vi "Read Next Message.vi"(7 "Ignore Error on Termination Message (F)":bool, 8 "error in (no error)":errorcluster, 9 "Termination List ([Exit])":string[](array[string])=["Exit"], 10 "timeout (1ms)":i32=1, 11 "Message Queue in":T3) -> (0 "error out":errorcluster, 1 "Message Value":string, 2 "Message Name":string, 3 "Message Queue out":T3, 4 "Message Attributes":T1, 5 "Exit Process":bool, 6 "Message":T2)   [LabVIEW 2013, in "AMC.lvlib"]
doc: "This VI returns the next message from the message queue passed in. If the returned message matches any of the message names listed in the Termination List the Exit Process indicator will return True. If no message is available on the queue within the Timeout limit, the VI returns with the Timed Out indicator set True."
uses:
  AMC.lvlib
  _SubVIs/TypeDefs/Message Queue.ctl
  _SubVIs/TypeDefs/Message.ctl
  Keyed Array/KeyedArray.ctl
  Keyed Array/Tools_KeyedArray.lvlib
panel:
  out "Timed Out":bool
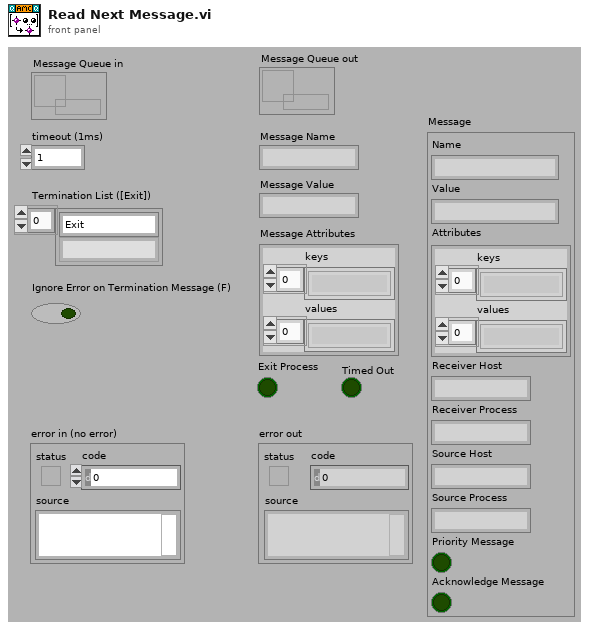
[diagram p1: front panel]
types:
  T1 = typedef "Tools_KeyedArray.lvlib/KeyedArray.ctl" = cluster{"keys":string[], "values":string[]}
  T2 = typedef "AMC.lvlib/Message.ctl" = cluster{"Name":string, "Value":string, "Attributes":T1, "Receiver Host":string, "Receiver Process":string, "Source Host":string, "Source Process":string, "Priority Message":bool, "Acknowledge Message":bool}
  T3 = typedef "AMC.lvlib/Message Queue.ctl" = refnum<queue>
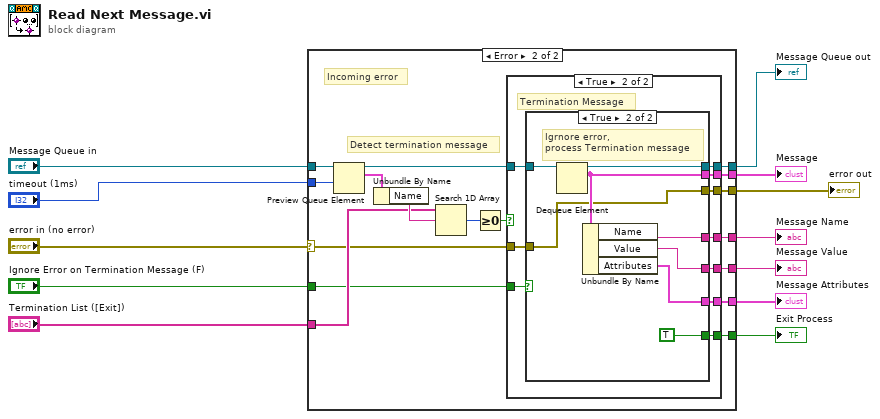
[diagram p0: block diagram]
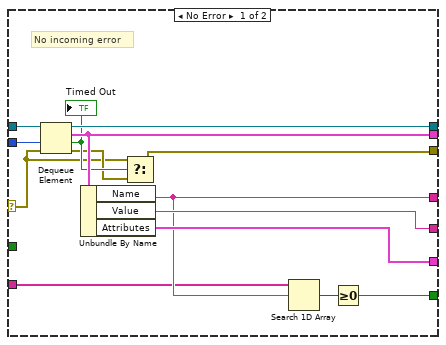
[diagram p2: hidden frame]
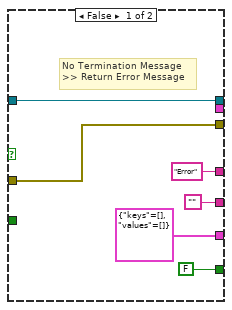
[diagram p3: hidden frame]
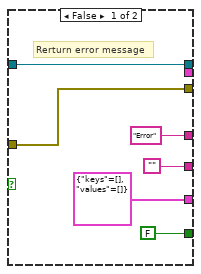
[diagram p4: hidden frame]
diagram:
  n1 = case shown="Error" "error in (no error)" {
    selector: "error in (no error)" -> [w13 w29]
    tunnel: "Message Queue in" -> [w26 w39]
    tunnel: [w25 w31] -> w10
    tunnel: [w20 w43] -> w12
    tunnel: "timeout (1ms)" -> [w24 w38]
    tunnel: [w14 w27] -> w11
    tunnel: [w22 w42] -> w9
    tunnel: [w23 w28] -> w8
    tunnel: [w21 w41] -> w7
    tunnel: "Termination List ([Exit])" -> [w19 w34]
    tunnel: [w17 w40] -> w6
    tunnel: "Ignore Error on Termination Message (F)" -> [_ w30]
    frame No Error {
      # "No incoming error"
      n2 = Dequeue Element(queue=w26, timeout in ms (-1)=w24, error in (no error)=w13) -> (queue out=w25:T3, element=w23:T2, timed out?=w16:bool, error out=w15:errorcluster)
      "Timed Out" <- w16
      n3 = Unbundle By Name(w23) -> ("Name"=w20:string, "Value"=w22:string, "Attributes"=w21:T1)
      n4 = Select(t=w13, s=w16, f=w15) -> (s? t:f=w14:errorcluster)
      n5 = Search 1D Array(1D array=w19, element=w20) -> (index of element=w18:i32)  [unwired: 1 out]
      n6 = Greater Or Equal To 0?(x=w18) -> (x >= 0?=w17:bool)
    }
    frame Error {
      # "Detect termination message"
      # "Incoming error"
      n7 = Preview Queue Element(queue=w39, timeout in ms (-1)=w38) -> (queue out=w32:T3, element=w37:T2)  [unwired: 1 in, 2 out]
      n8 = Unbundle By Name(w37) -> ("Name"=w35:string)
      n9 = Search 1D Array(1D array=w34, element=w35) -> (index of element=w36:i32)  [unwired: 1 out]
      n10 = Greater Or Equal To 0?(x=w36) -> (x >= 0?=w33:bool)
      n11 = case shown="True" w33 {
        tunnel: ["Error" w57] -> w43
        tunnel: ["" w56] -> w42
        tunnel: [T1 {"keys"=[], "values"=[]} ("Attributes") w55] -> w41
        tunnel: [FALSE w54] -> w40
        tunnel: [w45 w53] -> w31
        tunnel: w32 -> [w45 w59]
        tunnel: w30 -> [_ w58]
        tunnel: w29 -> [w44 w50]
        tunnel: [_ w52] -> w28
        tunnel: [w44 w51] -> w27
        frame False {
          # "No Termination Message\n>> Return Error Message"
        }
        frame True {
          # "Termination Message"
          n12 = case shown="True" w58 {
            tunnel: w59 -> [w61 w73]
            tunnel: ["Error" w70] -> w57
            tunnel: ["" w69] -> w56
            tunnel: [T1 {"keys"=[], "values"=[]} ("Attributes") w68] -> w55
            tunnel: [FALSE TRUE] -> w54
            tunnel: [w61 w66] -> w53
            tunnel: [_ w71] -> w52
            tunnel: [w60 w67] -> w51
            tunnel: w50 -> [w60 w67]
            frame False {
              # "Rerturn error message"
            }
            frame True {
              # "Igrnore error,\nprocess Termination message"
              n13 = Dequeue Element(queue=w73) -> (queue out=w66:T3, element=w71:T2)  [unwired: 2 in, 2 out]
              n14 = Unbundle By Name(w71) -> ("Name"=w70:string, "Value"=w69:string, "Attributes"=w68:T1)
            }
          }
        }
      }
    }
  }
  "Message Queue out" <- w10
  "Message Name" <- w12
  "error out" <- w11
  "Message Value" <- w9
  "Message" <- w8
  "Message Attributes" <- w7
  "Exit Process" <- w6
